vi "Write Max Points per Trace (all).vi"(8 "Error In":errorcluster, 10 "Max Points per Trace (all)":i32=-1, 11 "Trace Query Options Msg":refnum<class "Trace Query Options Msg.lvclass">) -> (0 "Error Out":errorcluster, 3 "Trace Query Options Msg":refnum<class "Trace Query Options Msg.lvclass">)   [LabVIEW 2020, in "BNT_DSCXtGraph.lvlib" / "Trace Query Options Msg.lvclass"]
uses:
  Trace Query Options Msg.lvclass
  Trace Query Options Msg.lvclass/Trace Query Options Msg.ctl
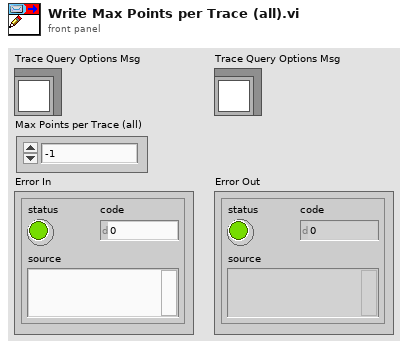
[diagram p1: front panel]
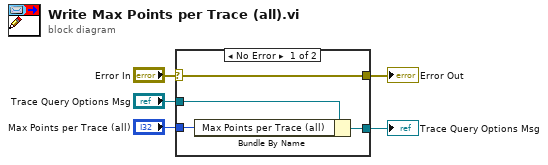
[diagram p0: block diagram]
diagram:
  n1 = case shown="No Error" "Error In" {
    selector: "Error In" -> [w9 w10]
    tunnel: [w9 w10] -> w5
    tunnel: [w7 w11] -> w3
    tunnel: "Trace Query Options Msg" -> [w8 w11]
    tunnel: "Max Points per Trace (all)" -> [w6 _]
    frame No Error {
      n2 = Bundle By Name(cluster=w8, "Max Points per Trace (all)"=w6) -> (w7:refnum<class "Trace Query Options Msg.lvclass">)
    }
    frame Error {
    }
  }
  "Trace Query Options Msg" <- w3
  "Error Out" <- w5
